vi "Test Inherited Test Filter Inherited Tests.vi"(8 "error in (no error)":errorcluster, 11 "Test Case In":refnum<class "Filter Test.lvclass">) -> (0 "error out":errorcluster, 3 "Test Case Out":refnum<class "Filter Test.lvclass">)   [LabVIEW 2020, in "Filter Test.lvclass"]
uses:
  Filter Test.lvclass
  C:/Program Files (x86)/National Instruments/LabVIEW 2020/vi.lib/Astemes/LUnit/Test Case.lvclass
  Test Doubles/Test Case Test Double/Test Case Test Double Child.lvclass
  Test Doubles/Test Case Test Double Parent/Test Case Test Double Parent.lvclass
  <vilib>/Astemes/LUnit/Test Case.lvclass/Test Case.ctl
  508a1887-a8d8-4322-8ddf-55304e69a97e.vi
  <vilib>/Astemes/LUnit/Append Pass Result.vi
  <vilib>/Astemes/LUnit/Append Fail Result.vi
  <vilib>/Astemes/LUnit/Describe Comparison.vi
  <vilib>/Astemes/LUnit/Compare Variants.vi
  <vilib>/Astemes/LUnit/Describe Variant.vi
  source/Support/Filters/Inherited Tests Filter/Inherited Tests Filter.lvclass
  source/API/LUnit Test Suite/LUnit Test Suite.lvclass
panel:
  out "List of Runnables":string[](array[string])
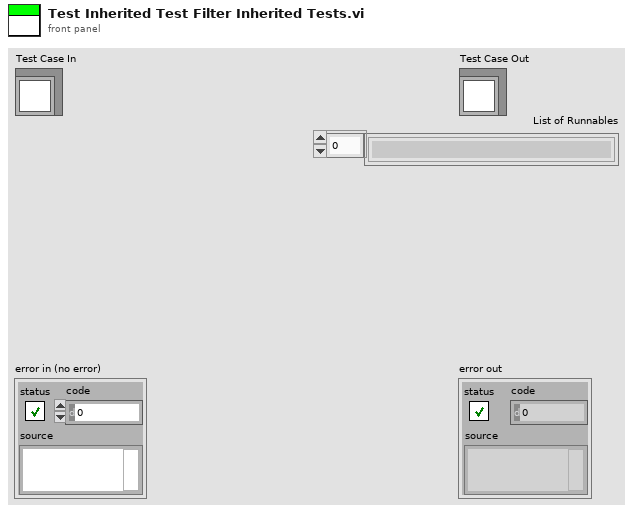
[diagram p1: front panel]
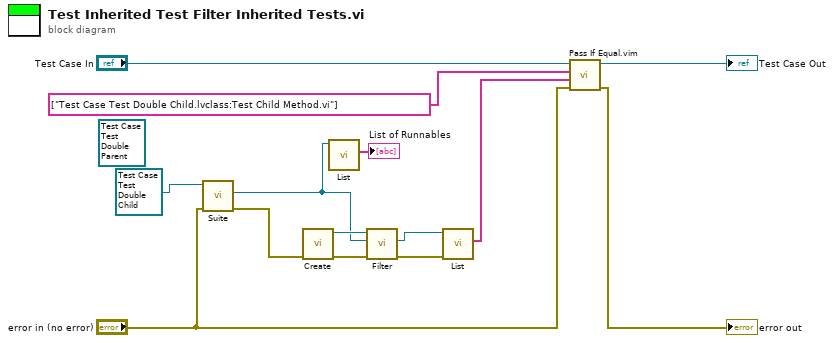
[diagram p0: block diagram]
diagram:
  (unwired) refnum<class "Test Case Test Double Parent.lvclass"> refnum ("Test Case Test Double Parent.lvclass")
  n1 = call-dynamic "Suite.vi"("error in (no error)"="error in (no error)", "LUnit Test Case in"=refnum<class "Test Case Test Double Child.lvclass"> refnum ("Test Case Test Double Child.lvclass")) -> ("error out"=w11:errorcluster, "LUnit Test Suite Out"=w3:refnum<class "LUnit Test Suite.lvclass">)  [unwired: 7 in, 1 out]
  n2 = call "Create.vi"("error in (no error)"=w11) -> ("error out"=w9:errorcluster, "Inherited Tests Filter"=w10:refnum<class "Inherited Tests Filter.lvclass">)  [unwired: 9 in]
  n3 = call "List.vi"("LUnit Test Suite In"=w3) -> ("List of Runnables"=→"List of Runnables":string[])  [unwired: 9 in, 1 out]
  n4 = call-dynamic "Filter.vi"("error in (no error)"=w9, "Test Suite"=w3, "Inherited Tests Filter In"=w10) -> ("error out"=w6:errorcluster, "Filtered Test Suite"=w7:refnum<class "LUnit Test Suite.lvclass">)  [unwired: 7 in]
  n5 = call "List.vi"("error in (no error)"=w6, "LUnit Test Suite In"=w7) -> ("List of Runnables"=w5:string[])  [unwired: 8 in, 1 out]
  n6 = call "Pass If Equal.vim"("error in (no error)"="error in (no error)", "Actual"=w5, "Expected"=string[] ["Test Case Test Double Child.lvclass:Test Child Method.vi"] ("List of Runnables"), "LUnit Test Case In"="Test Case In") -> ("error out"=→"error out":errorcluster, "LUnit Test Case Out"=→"Test Case Out":refnum<class "Filter Test.lvclass">)  [unwired: 6 in]
